vi "WSVCAP SHL FPGA LL SPI FIFO Manager - Pre and Post.vi"(0 "Word In":u16, 7 "timeout in ms (-1)":i32, 11 "error in (no error)":errorcluster, 13 "Operation":T1) -> (8 "Timed Out":bool, 10 "Word Out":u16, 15 "error out":errorcluster)   [LabVIEW 2017]
uses:
  Type Defs/WSVCAP SHL FIFO Operation Enum.ctl
  <vilib>/rvi/Emulation/niFpgaEmulationIsFPGAContextNoSignature.vi
  <vilib>/rvi/Emulation/niFpgaSctlEmulationGetInTimedLoop.vi
  <vilib>/rvi/errors/niFpgaSetErrorForExecOnDevCompSimple.vi
  <vilib>/rvi/eio/common/nirviEmuReportErrorAndStop.vi
  <vilib>/rvi/DataTransferAndStorage/Container/Common/niFpgaContainerGetUniqueNameForEmu.vi
  <vilib>/rvi/FIFO/Fifo_Resource/nirvififoEmulationSetSize.vi
  <vilib>/rvi/FIFO/Fifo_Resource/nirviFifoEmulationQueueMgr.vi
  <instcachedir>/0/nirviFifoEmulationQueueMgr_E5CAEC123FF24DC58D834DCA3CDAA9B5.lvgen/nirviFifoEmulationQueueMgr_E5CAEC123FF24DC58D834DCA3CDAA9B5_002.vi
  <vilib>/rvi/FIFO/Fifo_Resource/nirvififoEmulationDetermineInputValidOut.vi
  <vilib>/rvi/FIFO/Fifo_Resource/nirvififoEmulationCreateLock.vi
  <vilib>/rvi/Emulation/niFpgaProcessEmulError.vi
  <vilib>/rvi/FIFO/Fifo_Resource/nirvififoEmulationObtainLock.vi
  <vilib>/rvi/FIFO/Fifo_Resource/nirvififoEmulationReleaseLock.vi
  <vilib>/rvi/occurrence/nirviWaitOnOccurrenceBase.vi
  <vilib>/rvi/errors/nirviReportUnexpectedCaseInternalError.vi
  <vilib>/rvi/errors/nirviReportUnexpectedCaseInternalError (U32).vi
  <instcachedir>/0/nirviFifoEmulationQueueMgr_E5CAEC123FF24DC58D834DCA3CDAA9B5.lvgen/nirviFifoEmulationQueueMgr_E5CAEC123FF24DC58D834DCA3CDAA9B5_001.vi
  <vilib>/Utility/error.llb/Clear Errors.vi
  <vilib>/rvi/DataTransferAndStorage/Container/XNode/niFpgaContainer.xnode
  <vilib>/rvi/FIFO/Fifo_Resource/nirvififoEmulationWrite.vi
  <vilib>/rvi/FIFO/Fifo_Resource/nirvififoEmulationRead.vi
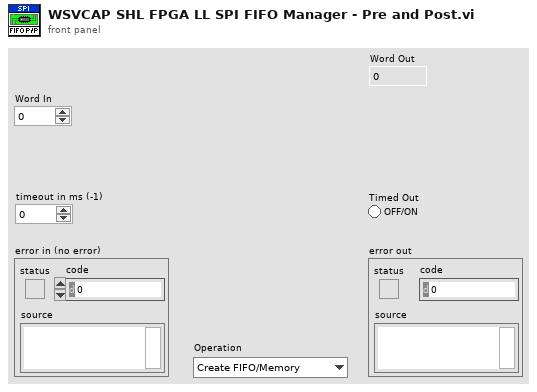
[diagram p1: front panel]
types:
  T1 = typedef "WSVCAP SHL FIFO Operation Enum.ctl" = enum16{"Create FIFO/Memory", "Get Write FIFO Status", "Get Read FIFO Status", "Put Element in Write", "Put Element in Read", "Get Element from Write", "Get Element from Read"}
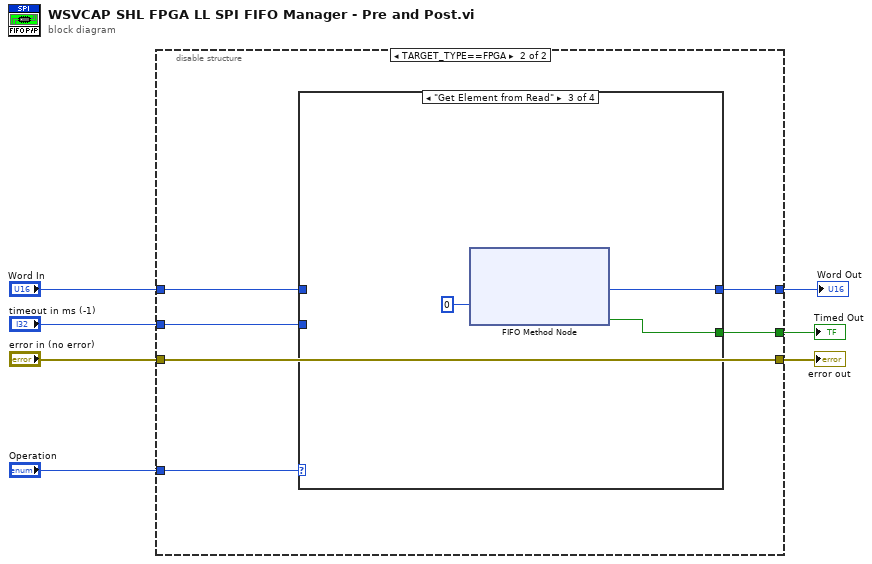
[diagram p0: block diagram]
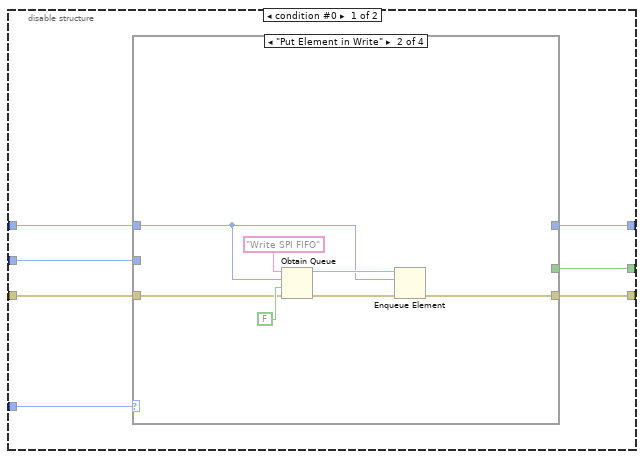
[diagram p2: hidden frame]
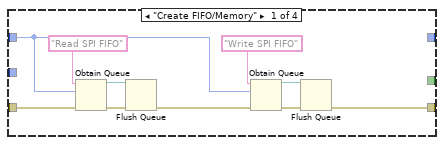
[diagram p3: hidden frame]
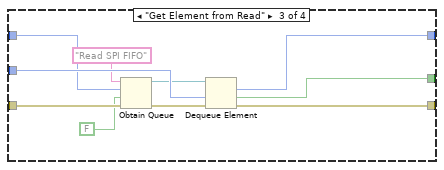
[diagram p4: hidden frame]
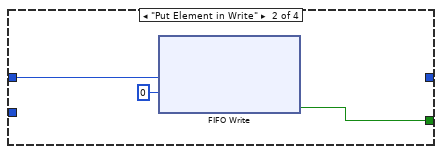
[diagram p7: hidden frame]
diagram:
  n1 = disable-structure shown="TARGET_TYPE==FPGA" {
    disable-tunnel: "Operation" -> [w14 w48]
    disable-tunnel: "error in (no error)" -> [w13 w43]
    disable-tunnel: [w12 w43] -> w5
    disable-tunnel: "Word In" -> [w11 w47]
    disable-tunnel: "timeout in ms (-1)" -> [w10 w46]
    disable-tunnel: [w9 w45] -> w2
    disable-tunnel: [w8 w44] -> w1
    frame condition #0 {
      n2 = case shown="\"Put Element in Write\"" w14 {
        tunnel: [w16 w26 w40 w42] -> w12
        tunnel: w13 -> [w23 w27 w38 w42]
        tunnel: w11 -> [w15 w25 w32 _]
        tunnel: w10 -> [_ _ w41 _]
        tunnel: [_ _ w39 _] -> w9
        tunnel: [_ _ w33 _] -> w8
        frame "Create FIFO/Memory" {
          n3 = Obtain Queue(name (unnamed)="Read SPI FIFO", element data type=w15, error in (no error)=w23) -> (queue out=w22:refnum<queue>, error out=w21:errorcluster)  [unwired: 2 in, 1 out]
          n4 = Flush Queue(queue=w22, error in (no error)=w21) -> (error out=w17:errorcluster)  [unwired: 2 out]
          n5 = Obtain Queue(name (unnamed)="Write SPI FIFO", element data type=w15, error in (no error)=w17) -> (queue out=w19:refnum<queue>, error out=w20:errorcluster)  [unwired: 2 in, 1 out]
          n6 = Flush Queue(queue=w19, error in (no error)=w20) -> (error out=w16:errorcluster)  [unwired: 2 out]
        }
        frame "Put Element in Write" {
          n7 = Obtain Queue(name (unnamed)="Write SPI FIFO", element data type=w25, create if not found? (T)=FALSE, error in (no error)=w27) -> (queue out=w30:refnum<queue>, error out=w31:errorcluster)  [unwired: 1 in, 1 out]
          n8 = Enqueue Element(queue=w30, element=w25, error in (no error)=w31) -> (error out=w26:errorcluster)  [unwired: 1 in, 2 out]
        }
        frame "Get Element from Read" {
          n9 = Obtain Queue(name (unnamed)="Read SPI FIFO", element data type=w32, create if not found? (T)=FALSE, error in (no error)=w38) -> (queue out=w35:refnum<queue>, error out=w37:errorcluster)  [unwired: 1 in, 1 out]
          n10 = Dequeue Element(queue=w35, timeout in ms (-1)=w41, error in (no error)=w37) -> (element=w33:u16, timed out?=w39:bool, error out=w40:errorcluster)  [unwired: 1 out]
        }
        frame Default {
        }
      }
    }
    frame condition #1 (active) {
      n11 = case shown="\"Get Element from Read\"" w48 {
        tunnel: w47 -> [_ w51 _ _]
        tunnel: w46 -> [_ _ _ _]
        tunnel: [_ w49 w53 _] -> w45
        tunnel: [_ _ w54 _] -> w44
        frame "Create FIFO/Memory" {
        }
        frame "Put Element in Write" {
          n12 = xnode "FIFO Write"("Element"=w51, "Timeout"=0) -> ("Timed Out?"=w49:bool)  [unwired: 1 in, 1 out]
        }
        frame "Get Element from Read" {
          n13 = xnode ("FIFO Method Node")("Timeout"=0) -> ("Element"=w54:u64, "Timed Out?"=w53:bool)  [unwired: 2 in, 2 out]
        }
        frame Default {
        }
      }
    }
  }
  "error out" <- w5
  "Timed Out" <- w2
  "Word Out" <- w1
